vi "PC Hard.vi"(11 "DataIn":T4) -> (3 "DataOut":T1)   [LabVIEW 2017]
doc: "SubVI criada para realizar o movimento do BOT em caso de partida Player 1 x PC no nível difícil"
uses:
  controls/DataIn.ctl
  controls/Tabuleiro.ctl
  controls/GameOption.ctl
  controls/DataOut.ctl
  controls/TabuleiroCoordenadas.ctl
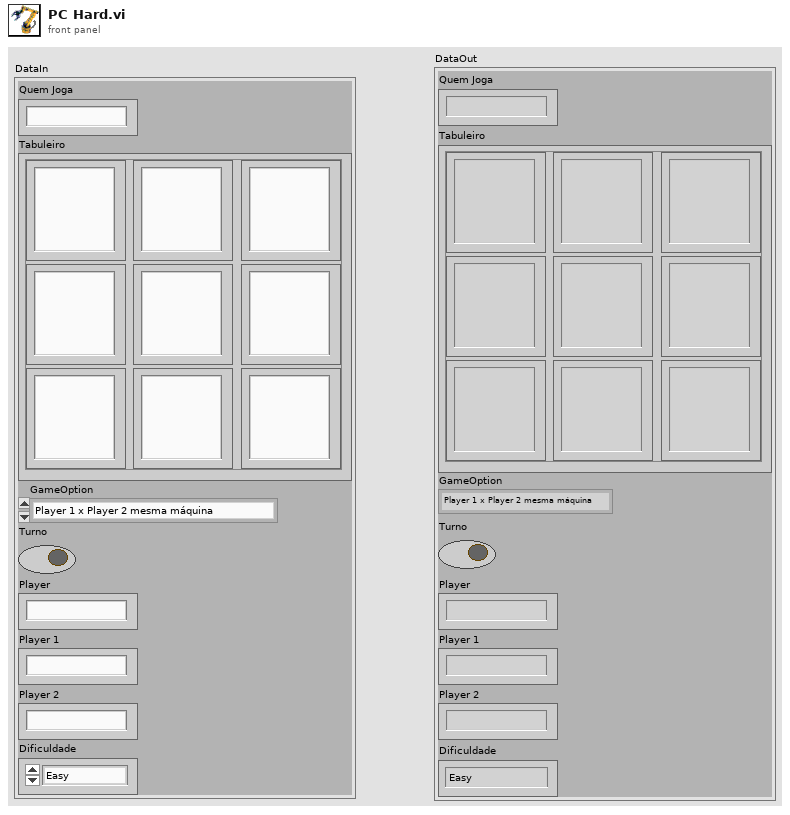
[diagram p1: front panel]
types:
  T1 = typedef "DataOut.ctl" = cluster{"Quem Joga":string, "Tabuleiro":T2, "GameOption":T3, "Turno":bool, "Player":string, "Player 1":string, "Player 2":string, "Dificuldade":enum16{"Easy", "Medium", "Hard"}}
  T2 = typedef "Tabuleiro.ctl" = cluster{"(0,0)":string, "(1,0)":string, "(0,1)":string, "(1,1)":string, "(2,0)":string, "(1,2)":string, "(2,2)":string, "(0,2)":string, "(2,1) ":string}
  T3 = typedef "GameOption.ctl" = enum16{"Player 1 x Player 2 mesma máquina", "Player 1 x Player 2 pela rede", "Player 1 x Computador", "Wait for Event", "Initialize", "Stop"}
  T4 = typedef "DataIn.ctl" = cluster{"Quem Joga":string, "Tabuleiro":T2, "GameOption":T3, "Turno":bool, "Player":string, "Player 1":string, "Player 2":string, "Dificuldade":enum16{"Easy", "Medium", "Hard"}}
  T5 = typedef "TabuleiroCoordenadas.ctl" = enum16{"0,0", "0,1", "0,2", "1,0", "1,1", "1,2", "2,0", "2,1", "2,2"}
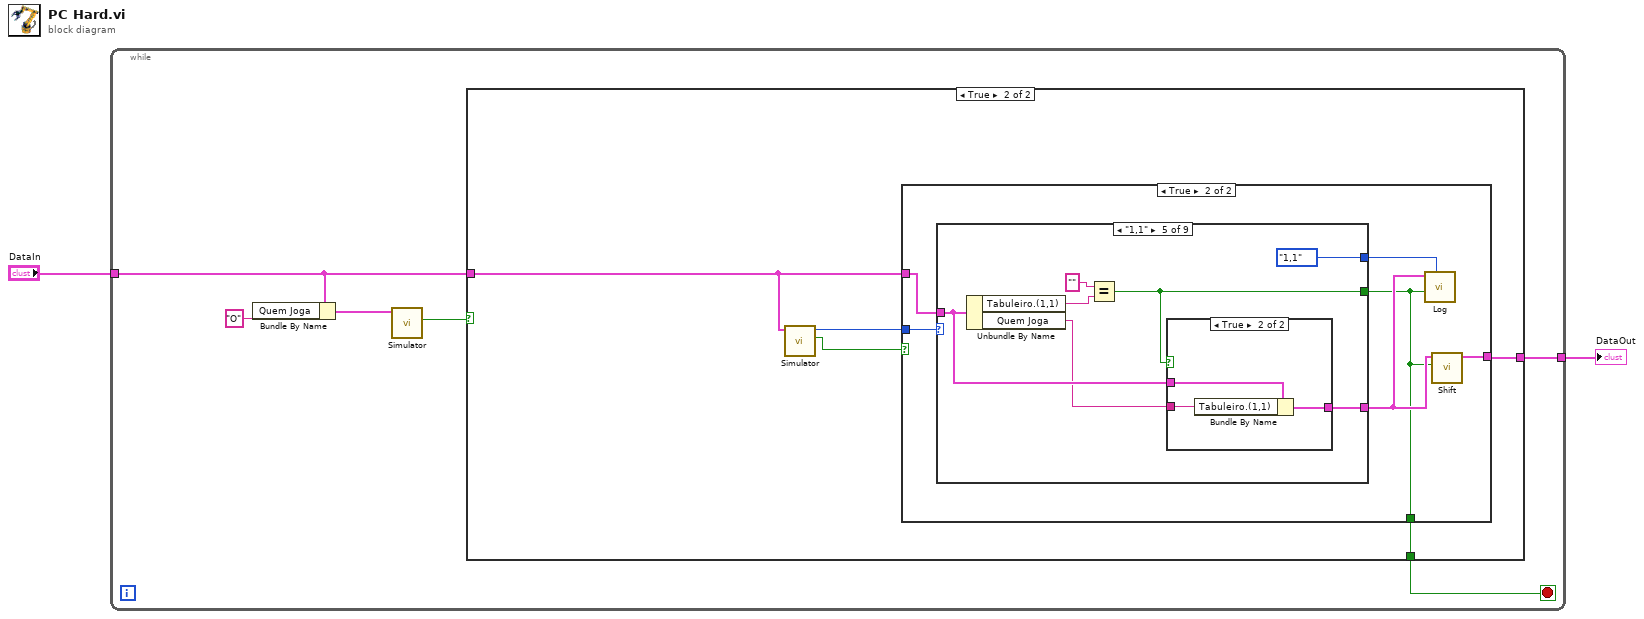
[diagram p0: block diagram]
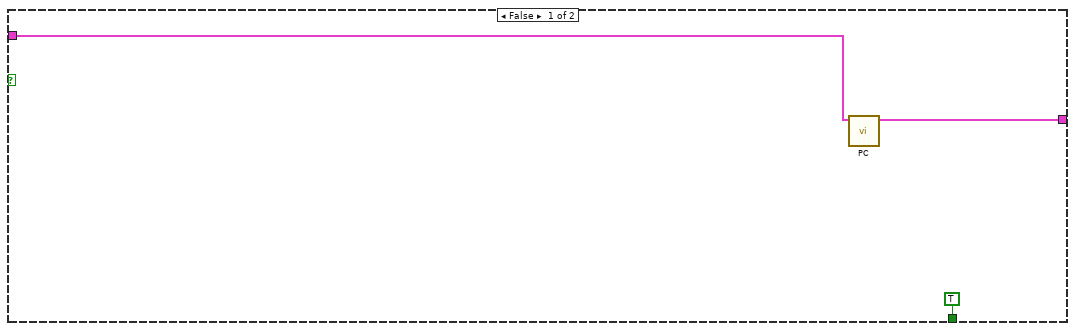
[diagram p2: hidden frame]
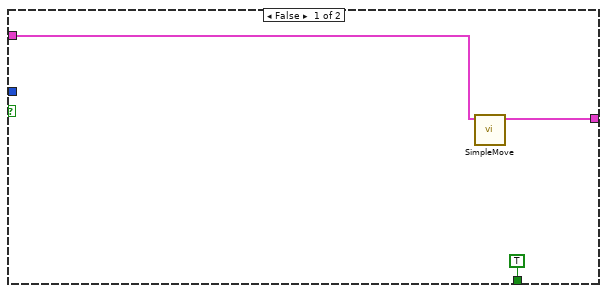
[diagram p3: hidden frame]
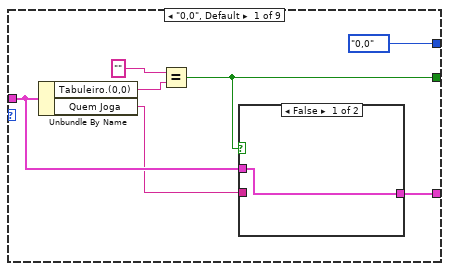
[diagram p4: hidden frame]
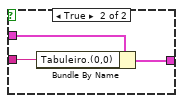
[diagram p5: hidden frame]
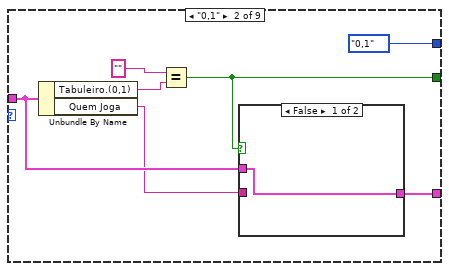
[diagram p6: hidden frame]
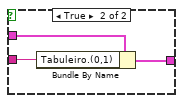
[diagram p7: hidden frame]
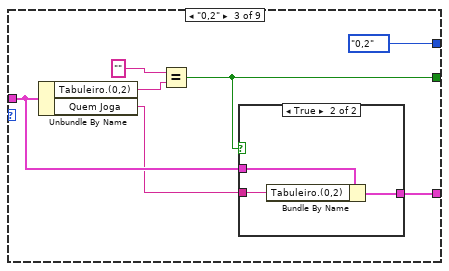
[diagram p8: hidden frame]
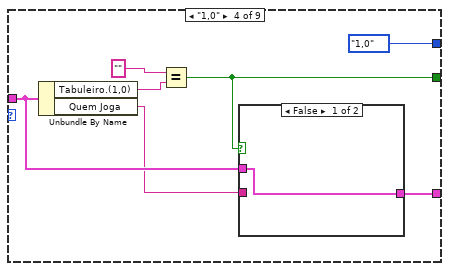
[diagram p10: hidden frame]
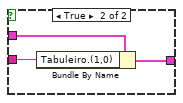
[diagram p11: hidden frame]
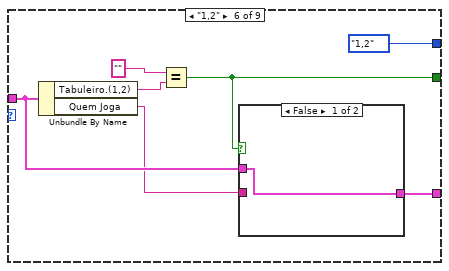
[diagram p13: hidden frame]
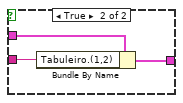
[diagram p14: hidden frame]
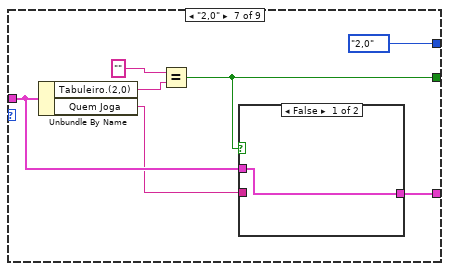
[diagram p15: hidden frame]
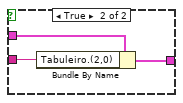
[diagram p16: hidden frame]
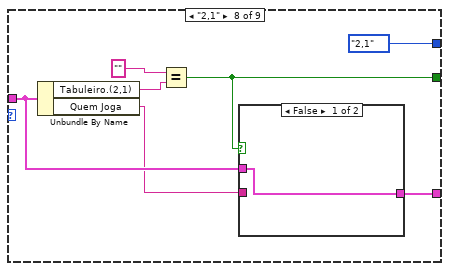
[diagram p17: hidden frame]
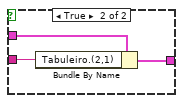
[diagram p18: hidden frame]
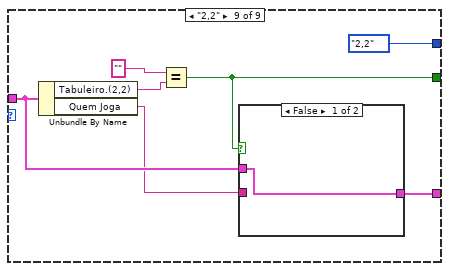
[diagram p19: hidden frame]
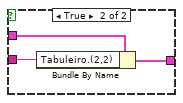
[diagram p20: hidden frame]
diagram:
  n1 = while {
    tunnel: [w8] -> w2
    tunnel: "DataIn" -> [w4]
    stop <- w3 stop-if-true
    n2 = Bundle By Name(cluster=w4, "Quem Joga"="O") -> (w5:T4)
    n3 = call "Simulator.vi"("DataIn"=w5) -> ("true = ganhou"=w7:bool)  [unwired: 9 in, 1 out]
    n4 = case shown="True" w7 {
      tunnel: [w11 w16] -> w8
      tunnel: w4 -> [w10 w13]
      tunnel: [TRUE w12] -> w3
      frame False {
        n5 = call "PC.vi"("DataIn"=w10) -> ("DataOut"=w11:T1)  [unwired: 10 in]
      }
      frame True {
        n6 = call "Simulator.vi"("DataIn"=w13) -> ("true = ganhou"=w14:bool, "Enum"=w15:T5)  [unwired: 9 in]
        n7 = case shown="True" w14 {
          tunnel: w15 -> [_ w25]
          tunnel: w13 -> [w18 w24]
          tunnel: [w19 w21] -> w16
          tunnel: [TRUE w20] -> w12
          frame False {
            n8 = call "SimpleMove.vi"("DataIn"=w18) -> ("DataOut"=w19:T1)  [unwired: 10 in]
          }
          frame True {
            n9 = case shown="\"1,1\"" w25 {
              tunnel: w24 -> [w29 w40 w51 w62 w73 w84 w95 w106 w117]
              tunnel: [w30 w41 w52 w63 w74 w85 w96 w107 w118] -> w20
              tunnel: [w27 w38 w49 w60 w71 w82 w93 w104 w115] -> w22
              tunnel: [TabuleiroCoordenadas."0,0" ("Enum") TabuleiroCoordenadas."0,1" ("Enum") TabuleiroCoordenadas."0,2" ("Enum") TabuleiroCoordenadas."1,0" ("Enum") TabuleiroCoordenadas."1,1" ("Enum") TabuleiroCoordenadas."1,2" ("Enum") TabuleiroCoordenadas."2,0" ("Enum") TabuleiroCoordenadas."2,1" ("Enum") TabuleiroCoordenadas."2,2" ("Enum")] -> w23
              frame "0,0", Default {
                n10 = Unbundle By Name(w29) -> ("Tabuleiro.(0,0)"=w32:string, "Quem Joga"=w28:string)
                n11 = Equal?(x="", y=w32) -> (x = y?=w30:bool)
                n12 = case shown="False" w30 {
                  tunnel: w29 -> [w33 w36]
                  tunnel: w28 -> [_ w35]
                  tunnel: [w33 w34] -> w27
                  frame False {
                  }
                  frame True {
                    n13 = Bundle By Name(cluster=w36, "Tabuleiro.(0,0)"=w35) -> (w34:T4)
                  }
                }
              }
              frame "0,1" {
                n14 = Unbundle By Name(w40) -> ("Tabuleiro.(0,1)"=w43:string, "Quem Joga"=w39:string)
                n15 = Equal?(x="", y=w43) -> (x = y?=w41:bool)
                n16 = case shown="False" w41 {
                  tunnel: w40 -> [w44 w47]
                  tunnel: w39 -> [_ w46]
                  tunnel: [w44 w45] -> w38
                  frame False {
                  }
                  frame True {
                    n17 = Bundle By Name(cluster=w47, "Tabuleiro.(0,1)"=w46) -> (w45:T4)
                  }
                }
              }
              frame "0,2" {
                n18 = Unbundle By Name(w51) -> ("Tabuleiro.(0,2)"=w54:string, "Quem Joga"=w50:string)
                n19 = Equal?(x="", y=w54) -> (x = y?=w52:bool)
                n20 = case shown="True" w52 {
                  tunnel: w51 -> [w55 w58]
                  tunnel: w50 -> [_ w57]
                  tunnel: [w55 w56] -> w49
                  frame False {
                  }
                  frame True {
                    n21 = Bundle By Name(cluster=w58, "Tabuleiro.(0,2)"=w57) -> (w56:T4)
                  }
                }
              }
              frame "1,0" {
                n22 = Unbundle By Name(w62) -> ("Tabuleiro.(1,0)"=w65:string, "Quem Joga"=w61:string)
                n23 = Equal?(x="", y=w65) -> (x = y?=w63:bool)
                n24 = case shown="False" w63 {
                  tunnel: w62 -> [w66 w69]
                  tunnel: w61 -> [_ w68]
                  tunnel: [w66 w67] -> w60
                  frame False {
                  }
                  frame True {
                    n25 = Bundle By Name(cluster=w69, "Tabuleiro.(1,0)"=w68) -> (w67:T4)
                  }
                }
              }
              frame "1,1" {
                n26 = Unbundle By Name(w73) -> ("Tabuleiro.(1,1)"=w76:string, "Quem Joga"=w72:string)
                n27 = Equal?(x="", y=w76) -> (x = y?=w74:bool)
                n28 = case shown="True" w74 {
                  tunnel: w73 -> [w77 w80]
                  tunnel: w72 -> [_ w79]
                  tunnel: [w77 w78] -> w71
                  frame False {
                  }
                  frame True {
                    n29 = Bundle By Name(cluster=w80, "Tabuleiro.(1,1)"=w79) -> (w78:T4)
                  }
                }
              }
              frame "1,2" {
                n30 = Unbundle By Name(w84) -> ("Tabuleiro.(1,2)"=w87:string, "Quem Joga"=w83:string)
                n31 = Equal?(x="", y=w87) -> (x = y?=w85:bool)
                n32 = case shown="False" w85 {
                  tunnel: w84 -> [w88 w91]
                  tunnel: w83 -> [_ w90]
                  tunnel: [w88 w89] -> w82
                  frame False {
                  }
                  frame True {
                    n33 = Bundle By Name(cluster=w91, "Tabuleiro.(1,2)"=w90) -> (w89:T4)
                  }
                }
              }
              frame "2,0" {
                n34 = Unbundle By Name(w95) -> ("Tabuleiro.(2,0)"=w98:string, "Quem Joga"=w94:string)
                n35 = Equal?(x="", y=w98) -> (x = y?=w96:bool)
                n36 = case shown="False" w96 {
                  tunnel: w95 -> [w99 w102]
                  tunnel: w94 -> [_ w101]
                  tunnel: [w99 w100] -> w93
                  frame False {
                  }
                  frame True {
                    n37 = Bundle By Name(cluster=w102, "Tabuleiro.(2,0)"=w101) -> (w100:T4)
                  }
                }
              }
              frame "2,1" {
                n38 = Unbundle By Name(w106) -> ("Tabuleiro.(2,1)"=w109:string, "Quem Joga"=w105:string)
                n39 = Equal?(x="", y=w109) -> (x = y?=w107:bool)
                n40 = case shown="False" w107 {
                  tunnel: w106 -> [w110 w113]
                  tunnel: w105 -> [_ w112]
                  tunnel: [w110 w111] -> w104
                  frame False {
                  }
                  frame True {
                    n41 = Bundle By Name(cluster=w113, "Tabuleiro.(2,1)"=w112) -> (w111:T4)
                  }
                }
              }
              frame "2,2" {
                n42 = Unbundle By Name(w117) -> ("Tabuleiro.(2,2)"=w120:string, "Quem Joga"=w116:string)
                n43 = Equal?(x="", y=w120) -> (x = y?=w118:bool)
                n44 = case shown="False" w118 {
                  tunnel: w117 -> [w121 w124]
                  tunnel: w116 -> [_ w123]
                  tunnel: [w121 w122] -> w115
                  frame False {
                  }
                  frame True {
                    n45 = Bundle By Name(cluster=w124, "Tabuleiro.(2,2)"=w123) -> (w122:T4)
                  }
                }
              }
            }
            n46 = call "Log.vi"("Enum Coordenadas"=w23, "Confirmação"=w20, "DataIn"=w22) -> ()  [unwired: 7 in, 2 out]
            n47 = call "Shift.vi"("Confirmação"=w20, "DataIn"=w22) -> ("DataOut"=w21:T1)  [unwired: 7 in, 2 out]
          }
        }
      }
    }
  }
  "DataOut" <- w2
